vi "Receive Message.vi"(0 "VISA Session In":refnum<visa-resource-name>="OXYMAT", 11 "error in (no error)":errorcluster) -> (4 "VISA Session Out":refnum<visa-resource-name>, 6 "Message Header":T1 {"Source Address" format="%.0x"; "Target Address" format="%.0x"}, 8 "Command echo":string, 10 "Response":string, 13 "Success":bool, 15 "error out":errorcluster)   [LabVIEW 2023, in "Siemens ELAN.lvlib"]
doc: "Lower-level VI which finds and parses a message, encoded using the Siemens ELAN protocol, received on the COM port specified by the VISA session. Returns the addressing and status info in a cluster, and any command/data response in two strings for further processing. Outputs only valid if 'Success' boolean indicates a complete message was found.\n\n$Revision:: 0 $\n$Modtime:: yy-mm-dd hh:mm $\n$Author:: Dboyd $"
uses:
  Siemens ELAN.lvlib
  Message Header.ctl
  Channel Status.ctl
panel:
  in  "Message Header":T1 {"Source Address" format="%.0x"; "Target Address" format="%.0x"}
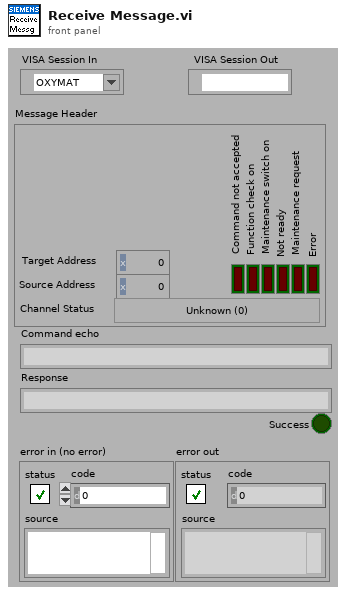
[diagram p1: front panel]
types:
  T1 = typedef "Siemens ELAN.lvlib/Message Header.ctl" = cluster{"Target Address":u8, "Source Address":u8, "Error":bool, "Maintenance request":bool, "Not ready":bool, "Maintenance switch on":bool, "Function check on":bool, "Command not accepted":bool, "Channel Status":T2}
  T2 = typedef "Siemens ELAN.lvlib/Channel Status.ctl" = enum8{"Unknown (0)", "Warm-up", "Pause", "Standby", "Measure", "Zero calibration", "Adjust component slope", "Unknown (7)", "Adjust curve dip", "Adjust linearization sensitivity", "Adjust temperature compensation", "Adjust pressure compensation", "Adjust linearization zero", "Adjust flow sensor", "Autocal", "Adjust phase", "Zero calibration of O2 sensor", "Synchronous zero calibration", "Purging for synchronous zero calibration", "Adjust analog output", "Adjust analog input", "Cleaning", "Unknown (>21)"}
  T3 = cluster{"unsigned byte array[0]":u8, "unsigned byte array[1]":u8, "unsigned byte array[2]":u8, "unsigned byte array[3]":u8}
  T4 = cluster{"Boolean array[0]":bool, "Boolean array[1]":bool, "Boolean array[2]":bool, "Boolean array[3]":bool, "Boolean array[4]":bool, "Boolean array[5]":bool}
  T5 = cluster{"unsigned byte array[0]":u8, "unsigned byte array[1]":u8, "Boolean array":cluster{"Boolean array[0]":bool, "Boolean array[1]":bool, "Boolean array[2]":bool, "Boolean array[3]":bool, "Boolean array[4]":bool, "Boolean array[5]":bool}, "unsigned byte array[3]":u8}
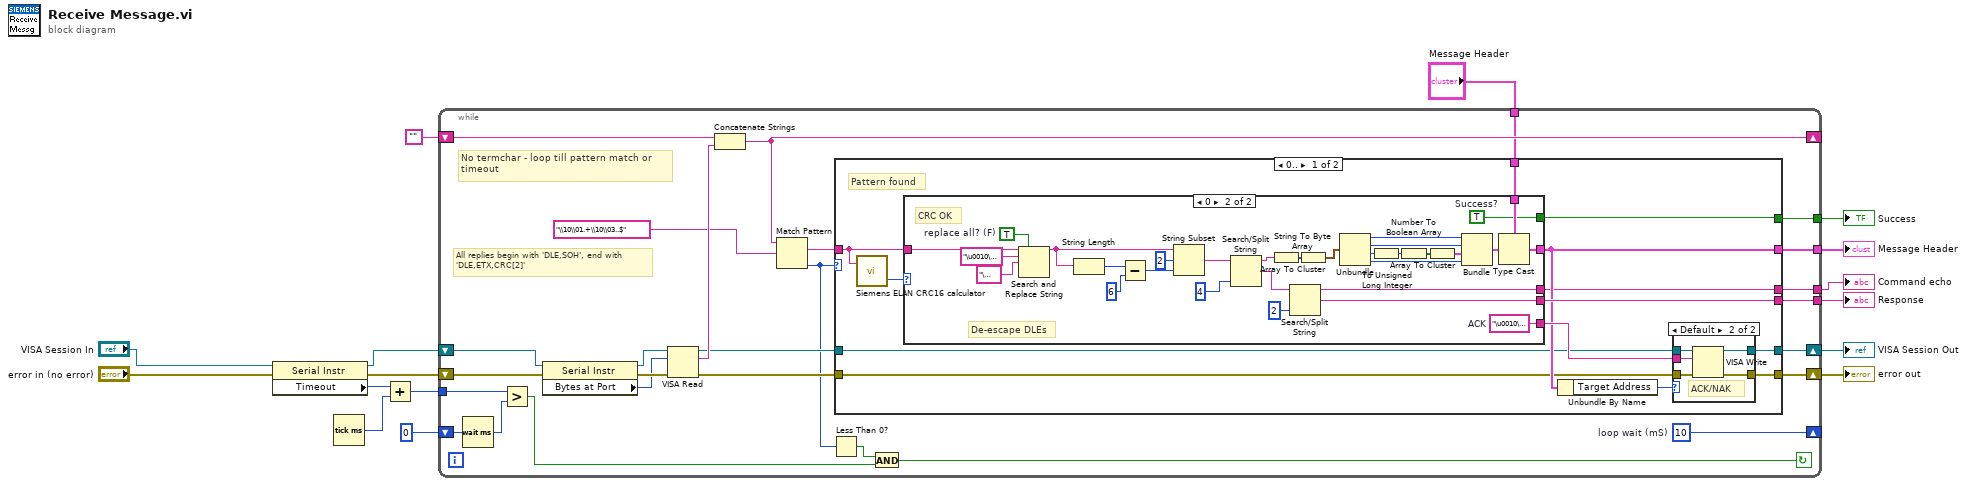
[diagram p0: block diagram]
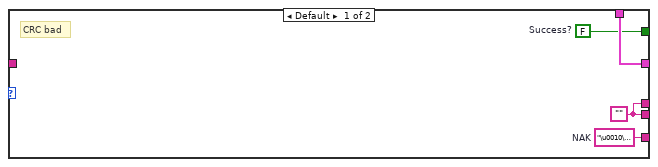
[diagram p3: hidden frame]
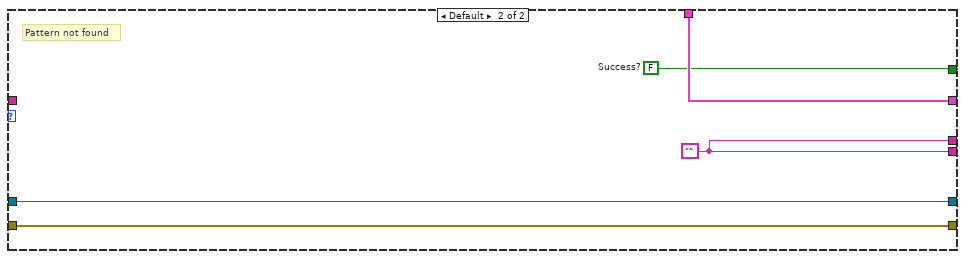
[diagram p4: hidden frame]
diagram:
  n1 = property class="Serial Instr"(reference="VISA Session In", error in="error in (no error)") -> (reference out=w15:refnum<visa-resource-name>, error out=w14:errorcluster, "Timeout"=w13:u32)
  n2 = Tick Count (ms)() -> (millisecond timer value=w12:u32)
  n3 = Add(x=w13, y=w12) -> (x+y=w11:u32)
  n4 = while {
    shift-right: [w33] -> _
    shift-left: "" -> [w36]
    shift-right: [w27] -> w7
    shift-left: w15 -> [w40]
    shift-right: [w26] -> w6
    shift-left: w14 -> [w41]
    tunnel: w11 -> [w42]
    shift-right: [w31] -> _
    shift-left: u32 0 ("milliseconds to wait") -> [w32]
    tunnel: "Message Header" -> [w24]
    tunnel: [w23] -> w8
    tunnel: [w22] -> w5
    tunnel: [w21] -> w4
    tunnel: [w17] -> w1
    stop <- w18 continue-if-true
    w31 = u32 10  # loop wait (mS)
    # "No termchar - loop till pattern match or\ntimeout"
    # "All replies begin with 'DLE,SOH', end with\n'DLE,ETX,CRC[2]'"
    n5 = Wait (ms)(milliseconds to wait=w32) -> (millisecond timer value=w43:u32)
    n6 = Greater?(x=w42, y=w43) -> (0:w30:bool)
    n7 = property class="Serial Instr"(reference=w40, error in=w41) -> (reference out=w38:refnum<visa-resource-name>, error out=w39:errorcluster, "Bytes at Port"=w37:u32)
    n8 = VISA Read(VISA resource name=w38, byte count=w37, error in (no error)=w39) -> (VISA resource name out=w29:refnum<visa-resource-name>, read buffer=w35:string, error out=w28:errorcluster)  [unwired: 1 out]
    n9 = Concatenate Strings(w36, w35) -> (w33:string)
    n10 = Match Pattern(string=w33, regular expression="\\10\\01.+\\10\\03..$") -> (match substring=w25:string, offset past match=w20:i32)  [unwired: 1 in, 2 out]
    n11 = Less Than 0?(x=w20) -> (x < 0?=w19:bool)
    n12 = case shown="0.." w20 {
      tunnel: w25 -> [w54 _]
      tunnel: w28 -> [w47 w100]
      tunnel: w29 -> [w48 w101]
      tunnel: [w51 w101] -> w27
      tunnel: [w53 w100] -> w26
      tunnel: w24 -> [w56 w102]
      tunnel: [w55 w98] -> w22
      tunnel: [w50 w102] -> w21
      tunnel: [w45 w99] -> w23
      tunnel: [w44 w98] -> w17
      frame 0.. {
        # "Pattern found"
        n13 = call "Siemens ELAN CRC16 calculator.vi"("Input String"=w54) -> ("CRC16 output"=w49:u16)  [unwired: 1 in, 1 out]
        n14 = case shown="0" w49 {
          tunnel: w54 -> [_ w74]
          tunnel: w56 -> [w66 w80]
          tunnel: [w66 w79] -> w50
          tunnel: [w64 w69] -> w55
          tunnel: [w67 w78] -> w52
          tunnel: [w65 w72] -> w45
          tunnel: [w64 w68] -> w44
          frame Default {
            w65 = FALSE  # Success?
            w64 = ""
            w67 = "\u0010\u0015"  # NAK
            # "CRC bad"
          }
          frame 0 {
            w72 = TRUE  # Success?
            w75 = TRUE  # replace all? (F)
            w78 = "\u0010\u0006"  # ACK
            # "De-escape DLEs"
            # "CRC OK"
            n15 = Search and Replace String(replace all?=w75, input string=w74, search string="\u0010\u0010", replace string="\u0010" ("replace string (\"\")")) -> (result string=w73:string)  [unwired: 4 in, 3 out]
            n16 = String Length(string=w73) -> (length=w92:i32)
            n17 = Subtract(x=w92, y=6) -> (x-y=w91:i32)
            n18 = String Subset(string=w73, offset (0)=2, length (rest)=w91) -> (substring=w89:string)
            n19 = Search/Split String(string=w89, offset (0)=4) -> (substring before match=w95:string, match + rest of string=w70:string)  [unwired: 1 in, 1 out]
            n20 = String To Byte Array(string=w95) -> (unsigned byte array=w97:u8[])
            n21 = Search/Split String(string=w70, offset (0)=2) -> (substring before match=w68:string, match + rest of string=w69:string)  [unwired: 1 in, 1 out]
            n22 = Array To Cluster(array=w97) -> (cluster=w94:T3)
            n23 = Unbundle(w94) -> ("unsigned byte array[0]"=w83:u8, "unsigned byte array[1]"=w84:u8, "unsigned byte array[2]"=w88:u8, "unsigned byte array[3]"=w85:u8)
            n24 = To Unsigned Long Integer(number=w88) -> (unsigned 32bit integer=w87:u32)
            n25 = Number To Boolean Array(number=w87) -> (Boolean array=w86:bool[])
            n26 = Array To Cluster(array=w86) -> (cluster=w82:T4)
            n27 = Bundle("unsigned byte array[0]"=w83, "unsigned byte array[1]"=w84, "Boolean array"=w82, "unsigned byte array[3]"=w85) -> (w81:T5)  [unwired: 1 in]
            n28 = Type Cast(type=w80, x=w81) -> (*(type *) &x=w79:T1)
          }
        }
        n29 = Unbundle By Name(w50) -> ("Target Address"=w46:u8)
        n30 = case shown="Default" w46 {
          tunnel: w47 -> [w57 w63]
          tunnel: w48 -> [w58 w62]
          tunnel: [w58 w61] -> w51
          tunnel: [w57 w60] -> w53
          tunnel: w52 -> [_ w59]
          frame 240..255 {
            # "Broadcast"
          }
          frame Default {
            # "ACK/NAK"
            n31 = VISA Write(VISA resource name=w62, write buffer=w59, error in (no error)=w63) -> (VISA resource name out=w61:refnum<visa-resource-name>, error out=w60:errorcluster)  [unwired: 1 out]
          }
        }
      }
      frame Default {
        w98 = ""
        w99 = FALSE  # Success?
        # "Pattern not found"
      }
    }
    n32 = And(x=w19, y=w30) -> (x .and. y?=w18:bool)
  }
  "VISA Session Out" <- w7
  "error out" <- w6
  "Response" <- w5
  "Message Header" <- w4
  "Success" <- w8
  "Command echo" <- w1
